vi "SpinSkillVSS.vi"(0 "object in":refnum<class "DefendGoalTacticVSS.lvclass">, 2 "Robot":refnum<class "Robot.lvclass">, 5 "error in (no error)":errorcluster) -> (14 "object out":refnum<class "DefendGoalTacticVSS.lvclass">, 16 "Robot 2":refnum<class "Robot.lvclass">, 19 "error out":errorcluster)   [LabVIEW 2023, in "DefendGoalTacticVSS.lvclass"]
uses:
  DefendGoalTacticVSS.lvclass
  Robot_class/Robot.lvclass
  DefendGoalTacticVSS.lvclass/DefendGoalTacticVSS.ctl
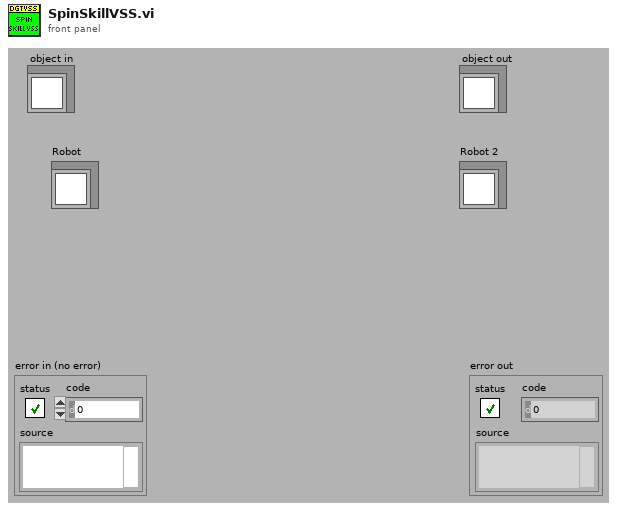
[diagram p1: front panel]
types:
  T1 = typedef "DefendGoalStates.ctl" = enum16{"Kick", "DefBallPos", "SpillSkin", "Exit"}
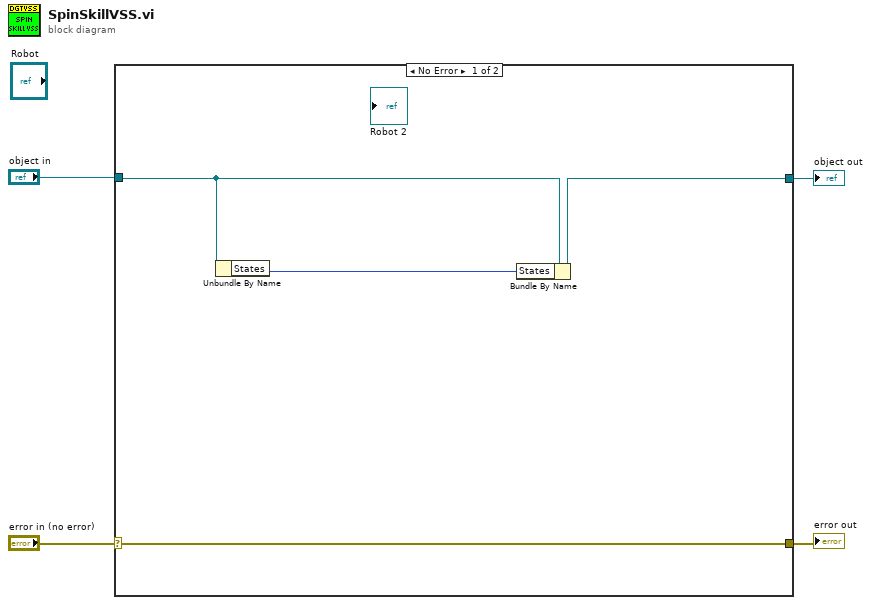
[diagram p0: block diagram]
diagram:
  n1 = case shown="No Error" "error in (no error)" {
    selector: "error in (no error)" -> [w7 w10]
    tunnel: [w7 w10] -> w3
    tunnel: [w5 w9] -> w1
    tunnel: "object in" -> [w6 w9]
    frame No Error {
      n2 = Unbundle By Name(w6) -> ("States"=w8:T1)
      n3 = Bundle By Name(cluster=w6, "States"=w8) -> (w5:refnum<class "DefendGoalTacticVSS.lvclass">)
    }
    frame Error {
    }
  }
  "error out" <- w3
  "object out" <- w1
